vi "Update Combobox Item Selection.vi"(10 "Object Config":T1, 11 "ComboBox in":refnum<vi>) -> ()   [LabVIEW 2017, in "Front Panel Publisher.lvlib" / "Web Front Panel.lvclass"]
uses:
  Web Front Panel.lvclass
  Controls/Enum - Control Display Mode.ctl
  Controls/FP Object Configuration.ctl
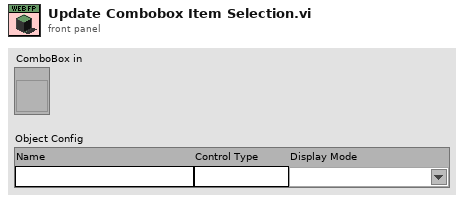
[diagram p1: front panel]
types:
  T1 = typedef "Front Panel Publisher.lvlib/Web Front Panel.lvclass/FP Object Configuration.ctl" = cluster{"Name":string, "Control Type":string, "Display Mode":string}
  T2 = typedef "Front Panel Publisher.lvlib/Web Front Panel.lvclass/Enum - Control Display Mode.ctl" = enum16{"Value Only", "Value and Visibility", "Boolean Value Only", "Boolean Value and Visibility", "Control is Image", "Image and Visibility"}
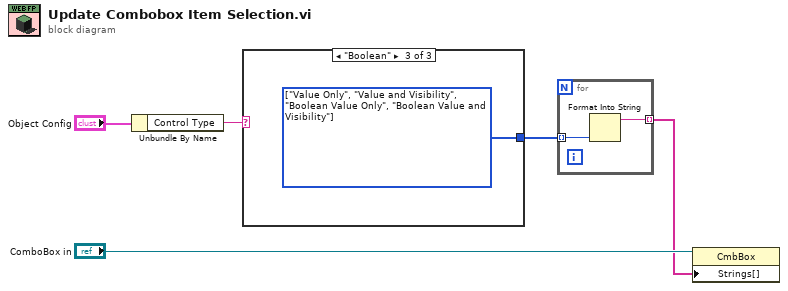
[diagram p0: block diagram]
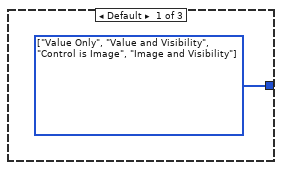
[diagram p2: hidden frame]
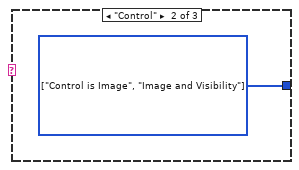
[diagram p3: hidden frame]
diagram:
  n1 = Unbundle By Name("Object Config") -> ("Control Type"=w4:string)
  n2 = case shown="\"Boolean\"" w4 {
    tunnel: [w6 w7 w8] -> w3
    frame Default {
      w6 = T2[] [enum."Value Only", enum."Value and Visibility", enum."Control is Image", enum."Image and Visibility"] items=["Value Only", "Value and Visibility", "Boolean Value Only", "Boolean Value and Visibility", "Control is Image", "Image and Visibility"]
    }
    frame "Control" {
      w7 = T2[] [enum."Control is Image", enum."Image and Visibility"] items=["Value Only", "Value and Visibility", "Boolean Value Only", "Boolean Value and Visibility", "Control is Image", "Image and Visibility"]
    }
    frame "Boolean" {
      w8 = T2[] [enum."Value Only", enum."Value and Visibility", enum."Boolean Value Only", enum."Boolean Value and Visibility"] items=["Value Only", "Value and Visibility", "Boolean Value Only", "Boolean Value and Visibility", "Control is Image", "Image and Visibility"]
    }
  }
  n3 = for {
    tunnel: w3 -> [w10] mode=indexing
    tunnel: [w9] -> w1 mode=indexing
    n4 = Format Into String(w10) -> (resulting string=w9:string)  [unwired: 3 in, 1 out]
  }
  n5 = property class="CmbBox"(reference="ComboBox in", "Strings[]"=w1) -> ()  [unwired: 1 in, 2 out]
